vi "LimeTimer.vi"(10 "Start?":bool) -> ()   [LabVIEW 2018]
uses:
  Robot Global Data.vi
  <vilib>/Rock Robotics/Network Tables/NT Read Number.vi
  <vilib>/Rock Robotics/Network Tables/NT Write Number.vi
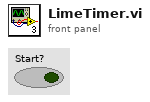
[diagram p1: front panel]
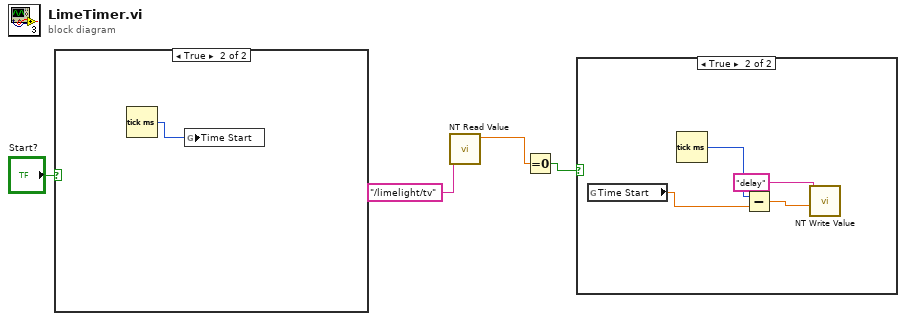
[diagram p0: block diagram]
diagram:
  n1 = case shown="True" "Start?" {
    frame False {
    }
    frame True {
      n2 = Tick Count (ms)() -> (millisecond timer value=w5:u32)
      n3 = global write "Robot Global Data.vi" "Time Start"(w5) -> ()
    }
  }
  n4 = call-poly <vilib>:"NT Read Value.vi"("Name"="/limelight/tv") -> ("Numeric"=w2:dbl)  [unwired: 9 in, 1 out]
  n5 = Equal To 0?(x=w2) -> (x = 0?=w3:bool)
  n6 = case shown="True" w3 {
    frame False {
    }
    frame True {
      n7 = global read "Robot Global Data.vi" "Time Start"() -> (w8:dbl)
      n8 = Tick Count (ms)() -> (millisecond timer value=w9:u32)
      n9 = Subtract(x=w9, y=w8) -> (x-y=w7:dbl)
      n10 = call-poly <vilib>:"NT Write Value.vi"("Numeric"=w7, "Name"="delay") -> ()  [unwired: 9 in, 1 out]
    }
  }
